vi "createTuplaEnDB.vi"(8 "error in":errorcluster, 11 "claseDB in":refnum<class "claseDB.lvclass">) -> (0 "error out":errorcluster, 3 "claseDB.lvclass":refnum<class "claseDB.lvclass">)   [LabVIEW 2014, in "claseDB.lvclass"]
uses:
  claseDB.lvclass
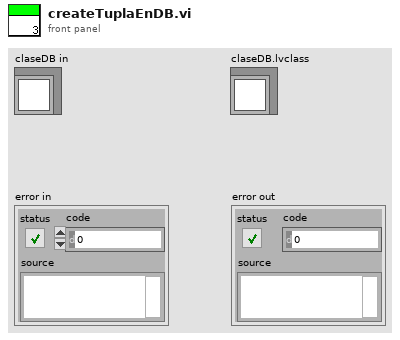
[diagram p1: front panel]
types:
  T1 = cluster{"objetoProduct":cluster{"idProduct":dbl, "od":string, "steelGrade":string, "lote":string, "dateCreate":timestamp, "idRecipe":dbl}, "objetoImage":cluster{"idImage":dbl, "camposDeMedicion":string, "dateCreate":timestamp}, "objetoRecipe":cluster{"idRecipe":dbl, "od":string, "steelGrade":string, "camposDeMedicion":string, "dateCreate":timestamp, "idStadistic":string}, "objetoStadistic":cluster{"idStadistic":dbl, "camposDeMedicion":string, "dateCreate":timestamp}, "objetoMetalRod":cluster{"idRod":dbl, "camposDeMedicion":string, "dateCreate":timestamp, "idProduct":dbl, "idImage":dbl}, "tableToUse":cluster{"useTableProduct":bool, "useTableImage":bool, "useTableRecipe":bool, "useTableStadistic":bool, "useTableMetalRod":bool}}
  T2 = cluster{"idProduct":dbl, "od":string, "steelGrade":string, "lote":string, "dateCreate":timestamp, "idRecipe":dbl}
  T3 = cluster{"idImage":dbl, "camposDeMedicion":string, "dateCreate":timestamp}
  T4 = cluster{"idRecipe":dbl, "od":string, "steelGrade":string, "camposDeMedicion":string, "dateCreate":timestamp, "idStadistic":string}
  T5 = cluster{"idStadistic":dbl, "camposDeMedicion":string, "dateCreate":timestamp}
  T6 = cluster{"idRod":dbl, "camposDeMedicion":string, "dateCreate":timestamp, "idProduct":dbl, "idImage":dbl}
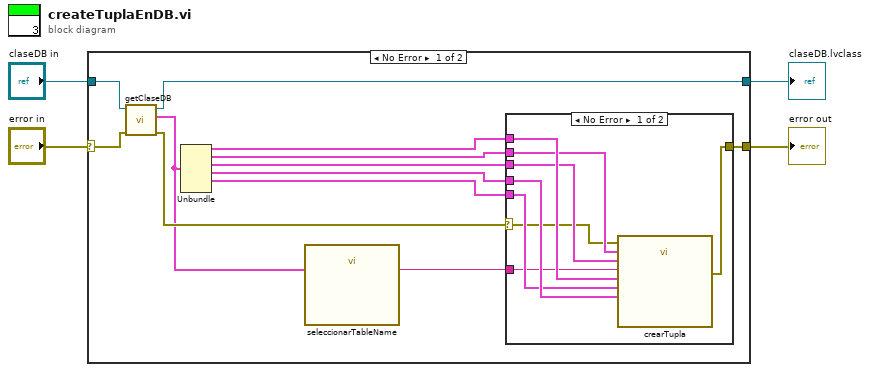
[diagram p0: block diagram]
diagram:
  n1 = case shown="No Error" "error in" {
    selector: "error in" -> [w8 w27]
    tunnel: "claseDB in" -> [w16 w26]
    tunnel: [w15 w27] -> w2
    tunnel: [w9 w26] -> w1
    frame No Error {
      n2 = call "getClaseDB.vi"("error in"=w8, "claseDB.lvclass"=w16) -> ("error out"=w6:errorcluster, "datosClaseDB"=w5:T1, "claseDB.lvclass 2"=w9:refnum<class "claseDB.lvclass">)  [unwired: 7 in]
      n3 = Unbundle(w5) -> ("objetoProduct"=w14:T2, "objetoImage"=w13:T3, "objetoRecipe"=w12:T4, "objetoStadistic"=w11:T5, "objetoMetalRod"=w10:T6)  [unwired: 1 out]
      n4 = call "seleccionarTableName.vi"("datosClaseDB in"=w5) -> ("tableNameOut"=w7:string)  [unwired: 10 in]
      n5 = case shown="No Error" w6 {
        selector: w6 -> [w17 w25]
        tunnel: [w24 w25] -> w15
        tunnel: w14 -> [w23 _]
        tunnel: w13 -> [w22 _]
        tunnel: w12 -> [w21 _]
        tunnel: w11 -> [w20 _]
        tunnel: w10 -> [w19 _]
        tunnel: w7 -> [w18 _]
        frame No Error {
          n6 = call "crearTupla.vi"("clusterMetalRodDataIn"=w19, "clusterProductDataIn"=w23, "clusterStadisticDataIn"=w20, "tableName"=w18, "clusterRecipeDataIn"=w21, "clusterImageDataIn"=w22, "error in"=w17) -> ("error out"=w24:errorcluster)  [unwired: 4 in]
        }
        frame Error {
        }
      }
    }
    frame Error {
    }
  }
  "error out" <- w2
  "claseDB.lvclass" <- w1
